vi "Teleop_Turret.vi"(11 "Joystick_IN":T1={"Pilot Left Joystick X"=0.015748031496062992, "Pilot Left Joystick Y"=-0.0, "Pilot A Button"=FALSE, "Pilot B Button"=FALSE, "Pilot X Button"=FALSE, "Pilot Y Button"=FALSE, "Pilot Left Bumper"=FALSE, "Pilot Right Bumper"=FALSE, "Pilot View Button"=FALSE, "Pilot Menu Button"=FALSE, "Pilot Left Joystick Press"=FALSE, "Pilot Right Joystick Press"=FALSE, "Pilot Left Trigger"=0.0, "Pilot Right Joystick X"=0.03937007874015748, "Pilot Right Joystick Y"=-0.015748031496062992, "Pilot Right Trigger"=0.0, "Copilot Left Joystick X"=0.0, "Copilot Left Joystick Y"=0.0, "Copilot A Button"=FALSE, "Copilot B Button"=FALSE, "Copilot X Button"=FALSE, "Copilot Y Button"=FALSE, "Copilot Left Bumper"=FALSE, "Copilot Right Bumper"=FALSE, "Copilot View Button"=FALSE, "Copilot Menu Button"=FALSE, "Copilot Left Joystick Press"=FALSE, "Copilot Right Joystick Press"=FALSE, "Copilot Left Trigger"=0.0, "Copilot Right Joystick X"=0.0, "Copilot Right Joystick Y"=0.0, "Copilot Right Trigger"=0.0, "Pilot D-pad North"=FALSE, "Pilot D-pad South"=FALSE, "Pilot D-pad East"=FALSE, "Pilot D-pad West"=FALSE, "Pilot D-pad NE "=FALSE, "Pilot D-pad SE"=FALSE, "Pilot D-pad SW"=FALSE, "Pilot D-pad NW"=FALSE, "CoPilot D-pad North"=TRUE, "CoPilot D-pad South"=FALSE, "CoPilot D-pad East"=FALSE, "CoPilot D-pad West"=FALSE, "CoPilot D-pad NE"=FALSE, "CoPilot D-pad SE"=FALSE, "CoPilot D-pad SW"=FALSE, "CoPilot D-pad NW"=FALSE, "Pilot Left Trigger Pressed"=FALSE, "Pilot Right Trigger Pressed"=FALSE, "CoPilot Left Trigger Pressed"=FALSE, "CoPilot Right Trigger Pressed"=FALSE}) -> ()   [LabVIEW 2019]
uses:
  Utility_VIs/Joystick_Controls.ctl
  Turret_Cluster.ctl
  Turret_Globals.vi
panel:
  in  "Turret_Spin_Power":dbl=0.7
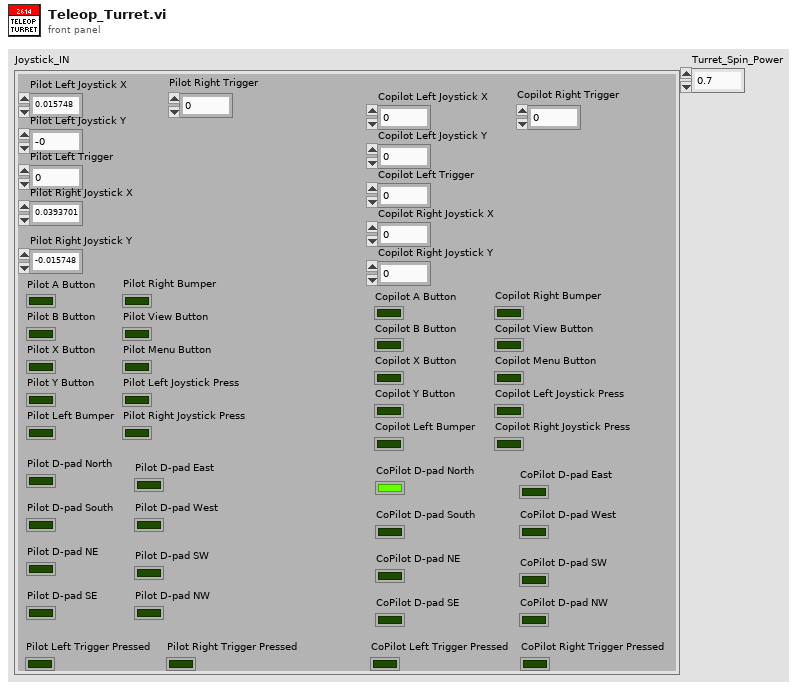
[diagram p1: front panel]
types:
  T1 = typedef "Joystick_Controls.ctl" = cluster{"Pilot Left Joystick X":dbl, "Pilot Left Joystick Y":dbl, "Pilot A Button":bool, "Pilot B Button":bool, "Pilot X Button":bool, "Pilot Y Button":bool, "Pilot Left Bumper":bool, "Pilot Right Bumper":bool, "Pilot View Button":bool, "Pilot Menu Button":bool, "Pilot Left Joystick Press":bool, "Pilot Right Joystick Press":bool, "Pilot Left Trigger":dbl, "Pilot Right Joystick X":dbl, "Pilot Right Joystick Y":dbl, "Pilot Right Trigger":dbl, "Copilot Left Joystick X":dbl, "Copilot Left Joystick Y":dbl, "Copilot A Button":bool, "Copilot B Button":bool, "Copilot X Button":bool, "Copilot Y Button":bool, "Copilot Left Bumper":bool, "Copilot Right Bumper":bool, "Copilot View Button":bool, "Copilot Menu Button":bool, "Copilot Left Joystick Press":bool, "Copilot Right Joystick Press":bool, "Copilot Left Trigger":dbl, "Copilot Right Joystick X":dbl, "Copilot Right Joystick Y":dbl, "Copilot Right Trigger":dbl, "Pilot D-pad North":bool, "Pilot D-pad South":bool, "Pilot D-pad East":bool, "Pilot D-pad West":bool, "Pilot D-pad NE ":bool, "Pilot D-pad SE":bool, "Pilot D-pad SW":bool, "Pilot D-pad NW":bool, "CoPilot D-pad North":bool, "CoPilot D-pad South":bool, "CoPilot D-pad East":bool, "CoPilot D-pad West":bool, "CoPilot D-pad NE":bool, "CoPilot D-pad SE":bool, "CoPilot D-pad SW":bool, "CoPilot D-pad NW":bool, "Pilot Left Trigger Pressed":bool, "Pilot Right Trigger Pressed":bool, "CoPilot Left Trigger Pressed":bool, "CoPilot Right Trigger Pressed":bool}
  T2 = typedef "Turret_Cluster.ctl" = cluster{"Control_State":enum16{"Manual_PercentVoltage", "Manual_SpeedControl", "Auto_Targeting", "Position"}, "Spin_Power":dbl, "Flywheel_Power":dbl, "Going_To_Position":bool}
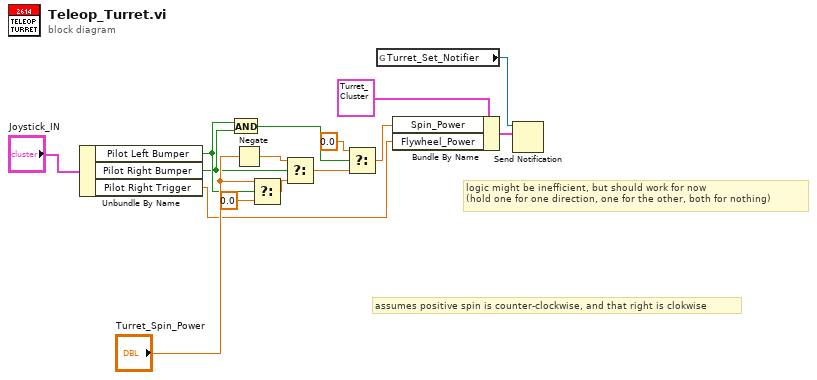
[diagram p0: block diagram]
diagram:
  # "logic might be inefficient, but should work for now\n(hold one for one direction, one for the other, both for nothing)"
  # "assumes positive spin is counter-clockwise, and that right is clokwise"
  n1 = Unbundle By Name("Joystick_IN") -> ("Pilot Left Bumper"=w7:bool, "Pilot Right Bumper"=w2:bool, "Pilot Right Trigger"=w1:dbl)
  n2 = And(x=w7, y=w2) -> (x .and. y?=w6:bool)
  n3 = Negate(x="Turret_Spin_Power") -> (-x=w9:dbl)
  n4 = Select(t="Turret_Spin_Power", s=w7, f=0.0) -> (s? t:f=w11:dbl)
  n5 = Select(t=w9, s=w2, f=w11) -> (s? t:f=w5:dbl)
  n6 = Select(t=0.0, s=w6, f=w5) -> (s? t:f=w3:dbl)
  n7 = global read "Turret_Globals.vi" "Turret_Set_Notifier"() -> (w14:refnum<notifier>)
  n8 = Bundle By Name(cluster=T2 {"Control_State"=enum."Manual_PercentVoltage", "Spin_Power"=0.0, "Flywheel_Power"=0.0, "Going_To_Position"=FALSE} ("notification"), "Spin_Power"=w3, "Flywheel_Power"=w1) -> (w12:T2)
  n9 = Send Notification(notification=w12, notifier=w14) -> ()  [unwired: 1 in, 2 out]
